vi "Generate Pattern String.vi"(10 "Options (Default)":T1, 11 "Part List":T2[](array[typedef])) -> (3 "Result":string)   [LabVIEW 2020, in "Stream.lvlib" / "URLPattern.lvclass"]
uses:
  URLPattern.lvclass
  Pattern Part.ctl
  Pattern Part Type.ctl
  Pattern Part Modifier.ctl
  Pattern String Options.ctl
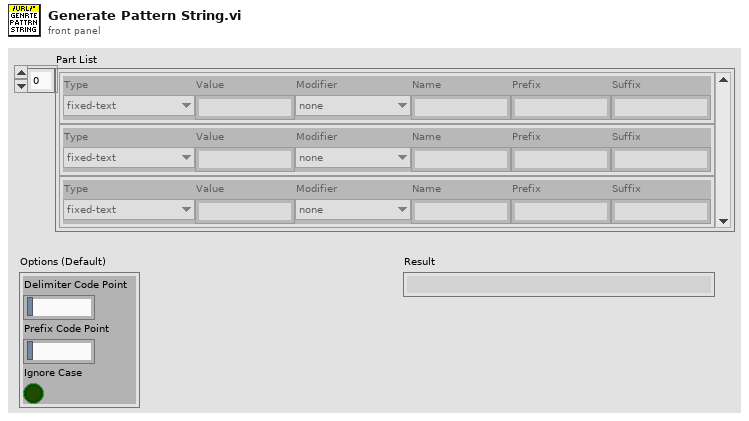
[diagram p1: front panel]
types:
  T1 = typedef "Stream.lvlib/URLPattern.lvclass/Pattern String Options.ctl" = cluster{"Delimiter Code Point":string, "Prefix Code Point":string, "Ignore Case":bool}
  T2 = typedef "Stream.lvlib/URLPattern.lvclass/Pattern Part.ctl" = cluster{"Type":T3, "Value":string, "Modifier":T4, "Name":string, "Prefix":string, "Suffix":string}
  T3 = typedef "Stream.lvlib/URLPattern.lvclass/Pattern Part Type.ctl" = enum16{"fixed-text", "regexp", "segment-wildcard", "full-wildcard"}
  T4 = typedef "Stream.lvlib/URLPattern.lvclass/Pattern Part Modifier.ctl" = enum16{"none", "optional", "zero-or-more", "one-or-more"}
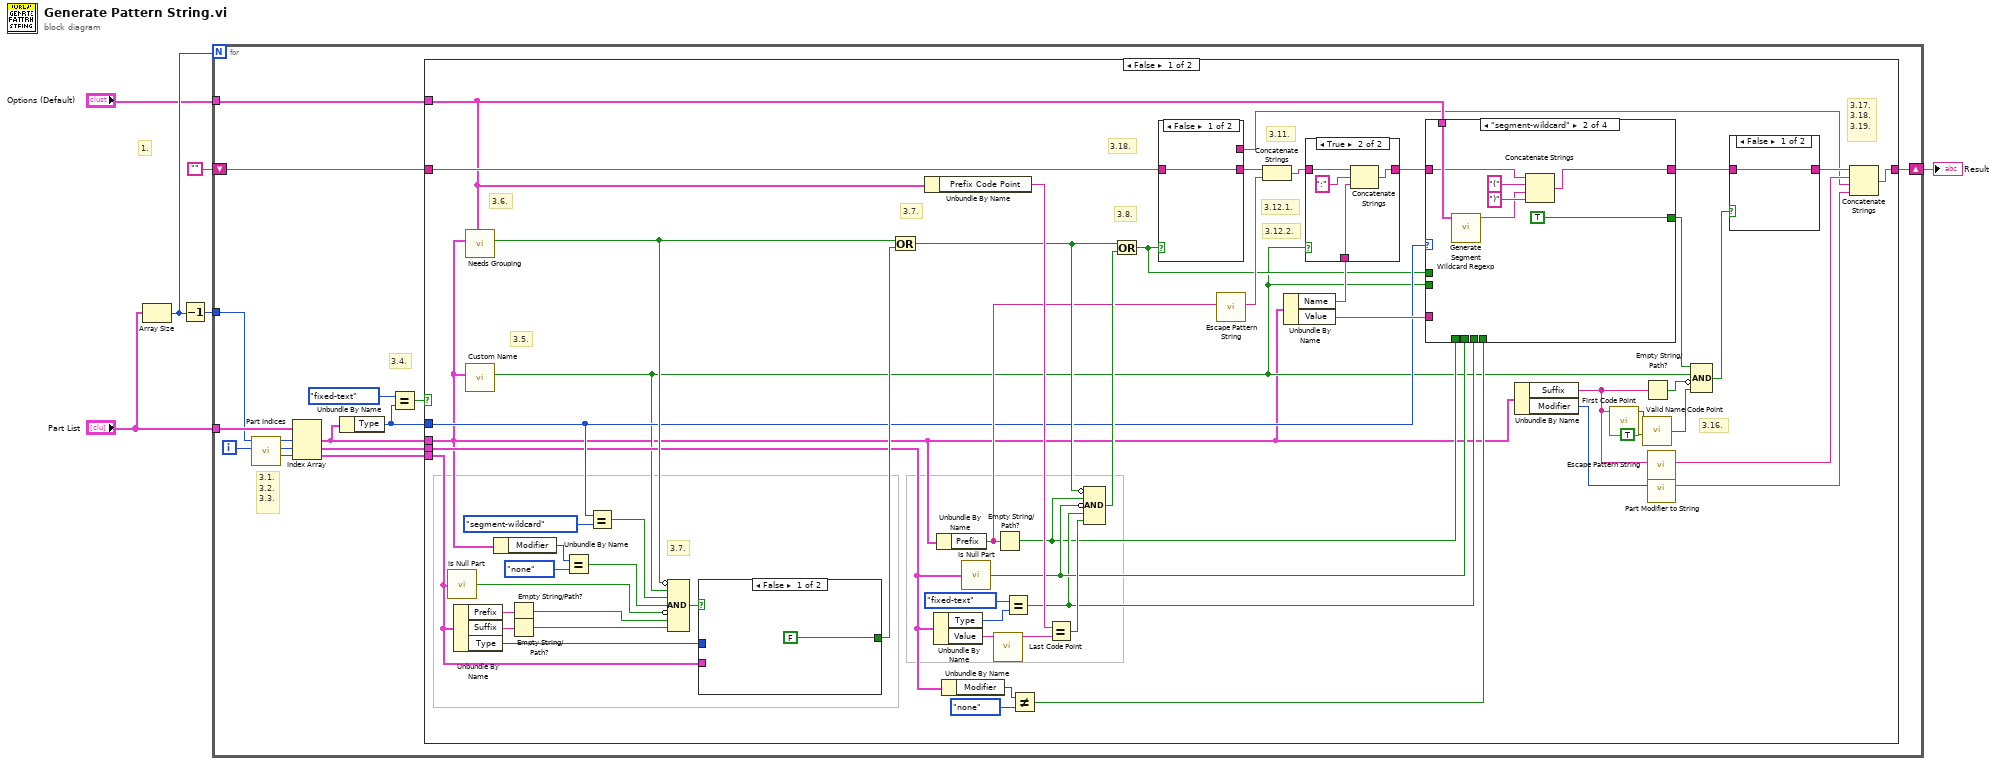
[diagram p0: block diagram]
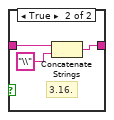
[diagram p2: hidden frame]
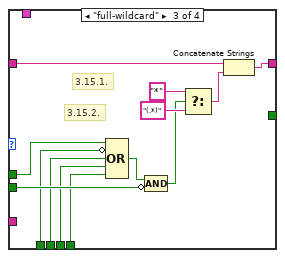
[diagram p4: hidden frame]
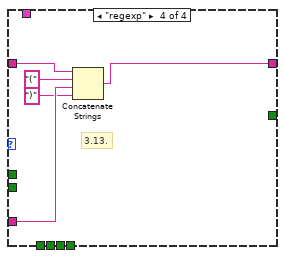
[diagram p5: hidden frame]
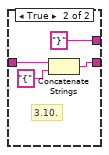
[diagram p7: hidden frame]
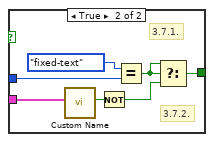
[diagram p8: hidden frame]
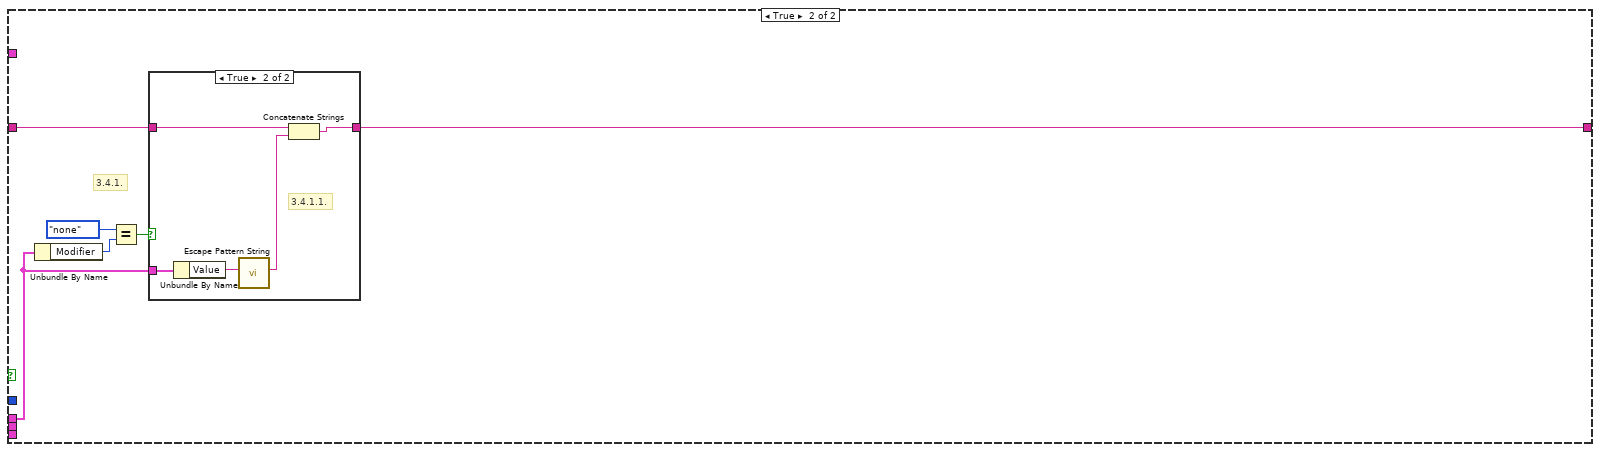
[diagram p9: hidden frame]
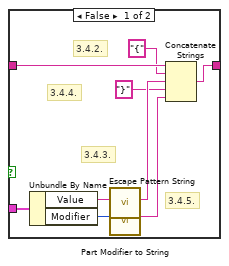
[diagram p10: hidden frame]
diagram:
  # "1."
  n1 = Array Size(array="Part List") -> (size(s)=w4:i32)
  n2 = Decrement(x=w4) -> (x-1=w3:i32)
  n3 = for {
    N: w4 -> [_]
    shift-right: [w8] -> w1
    shift-left: "" -> [w9]
    tunnel: "Part List" -> [w21]
    tunnel: w3 -> [w16]
    tunnel: "Options (Default)" -> [w10]
    i -> [w17]
    # "3.4."
    # "3.1.\n3.2.\n3.3."
    n4 = call "Part Indices.vi"("i"=w17, "Last Index"=w16) -> ("Next Index"=w18:i32, "Prev Index"=w19:i32, "Index"=w20:i32)  [unwired: 7 in]
    n5 = Index Array(array=w21, index #1=w20, index #2=w19, index #3=w18) -> (element #1=w13:T2, element #2=w12:T2, element #3=w11:T2)
    n6 = Unbundle By Name(w13) -> ("Type"=w7:T3)
    n7 = Equal?(x=Pattern_Part_Type."fixed-text", y=w7) -> (x = y?=w14:bool)
    n8 = case shown="False" w14 {
      tunnel: w13 -> [w35 w129]
      tunnel: w12 -> [w43 _]
      tunnel: w11 -> [w64 _]
      tunnel: w10 -> [w46 _]
      tunnel: w9 -> [w56 w128]
      tunnel: [w22 w127] -> w8
      tunnel: w7 -> [w47 _]
      frame False {
        # "3.18."
        # "3.17.\n3.18.\n3.19."
        # "3.16."
        # "3.12.2."
        # "3.12.1."
        # "3.11."
        # "3.8."
        # "3.7."
        # "3.7."
        # "3.6."
        # "3.5."
        n9 = call "Is Null Part.vi"("Pattern Part"=w64) -> ("Null Part"=w71:bool)
        n10 = Unbundle By Name(w64) -> ("Prefix"=w77:string, "Suffix"=w76:string, "Type"=w67:T3)
        n11 = call "Needs Grouping.vi"("Pattern String Options"=w46, "Pattern Part"=w35) -> ("Needs Grouping"=w66:bool)  [unwired: 9 in]
        n12 = call "Custom Name.vi"("Pattern Part"=w35) -> ("Custom Name?"=w36:bool)  [unwired: 10 in]
        n13 = Unbundle By Name(w35) -> ("Modifier"=w74:T4)
        n14 = Empty String/Path?(string/path=w77) -> (empty?=w70:bool)
        n15 = Empty String/Path?(string/path=w76) -> (empty?=w69:bool)
        n16 = Equal?(x=w74, y=Pattern_Part_Modifier."none") -> (x = y?=w72:bool)
        n17 = Equal?(x=w47, y=Pattern_Part_Type."segment-wildcard" ("x")) -> (x = y?=w48:bool)
        n18 = Compound Arithmetic op=AND(invert w66, w36, w48, w72, invert w71, w70, w69) -> (w68:bool)
        n19 = case shown="False" w68 {
          tunnel: w67 -> [_ w126]
          tunnel: w64 -> [_ w125]
          tunnel: [FALSE w120] -> w65
          frame False {
          }
          frame True {
            # "3.7.2."
            # "3.7.1."
            n20 = call "Custom Name.vi"("Pattern Part"=w125) -> ("Custom Name?"=w122:bool)  [unwired: 10 in]
            n21 = Not(x=w122) -> (.not. x?=w121:bool)
            n22 = Equal?(x=Pattern_Part_Type."fixed-text" ("y"), y=w126) -> (x = y?=w123:bool)
            n23 = Select(t=w123, s=w123, f=w121) -> (s? t:f=w120:bool)
          }
        }
        n24 = Or(x=w66, y=w65) -> (x .or. y?=w58:bool)
        n25 = Unbundle By Name(w46) -> ("Prefix Code Point"=w78:string)
        n26 = Unbundle By Name(w43) -> ("Type"=w63:T3, "Value"=w61:string)
        n27 = Unbundle By Name(w35) -> ("Prefix"=w55:string)
        n28 = Unbundle By Name(w43) -> ("Modifier"=w42:T4)
        n29 = call "Is Null Part.vi"("Pattern Part"=w43) -> ("Null Part"=w45:bool)
        n30 = call "Last Code Point.vi"("String"=w61) -> ("Last Code Point"=w60:string)  [unwired: 10 in]
        n31 = Empty String/Path?(string/path=w55) -> (empty?=w38:bool)
        n32 = Equal?(x=Pattern_Part_Type."fixed-text", y=w63) -> (x = y?=w44:bool)
        n33 = Not Equal?(x=w42, y=Pattern_Part_Modifier."none") -> (x != y?=w40:bool)
        n34 = Equal?(x=w78, y=w60) -> (x = y?=w59:bool)
        n35 = Compound Arithmetic op=AND(invert w58, w38, invert w45, w44, w59) -> (w57:bool)
        n36 = Or(x=w58, y=w57) -> (x .or. y?=w39:bool)
        n37 = case shown="False" w39 {
          tunnel: w56 -> [w114 w118]
          tunnel: [w114 w116] -> w54
          tunnel: [_ "}" ("string")] -> w25
          frame False {
          }
          frame True {
            # "3.10."
            n38 = Concatenate Strings(w118, "{" ("string")) -> (w116:string)
          }
        }
        n39 = call "Escape Pattern String.vi"("Input"=w55) -> ("Result"=w53:string)  [unwired: 10 in]
        n40 = Concatenate Strings(w54, w53) -> (w52:string)
        n41 = Unbundle By Name(w35) -> ("Name"=w51:string, "Value"=w49:string)
        n42 = case shown="True" w36 {
          tunnel: w52 -> [w109 w113]
          tunnel: [w109 w111] -> w50
          tunnel: w51 -> [_ w110]
          frame False {
          }
          frame True {
            n43 = Concatenate Strings(w113, ":" ("string"), w110) -> (w111:string)
          }
        }
        n44 = case shown="\"segment-wildcard\"" w47 {
          tunnel: w50 -> [w83 w87 w102 w108]
          tunnel: w49 -> [_ _ _ w106]
          tunnel: [w83 w85 w98 w104] -> w30
          tunnel: w46 -> [_ w90 _ _]
          tunnel: w36 -> [_ _ w103 _]
          tunnel: w45 -> [_ _ w96 _]
          tunnel: w44 -> [_ _ w95 _]
          tunnel: w40 -> [_ _ w94 _]
          tunnel: w39 -> [_ _ w93 _]
          tunnel: w38 -> [_ _ w92 _]
          tunnel: [_ TRUE _ _] -> w37
          frame Default {
          }
          frame "segment-wildcard" {
            n45 = call "Generate Segment Wildcard Regexp.vi"("Options"=w90) -> ("Segment Wildcard Regexp"=w86:string)  [unwired: 10 in]
            n46 = Concatenate Strings(w87, "(" ("string"), w86, ")" ("string")) -> (w85:string)
          }
          frame "full-wildcard" {
            # "3.15.2."
            # "3.15.1."
            n47 = Compound Arithmetic op=OR(w93, invert w92, w96, w95, w94) -> (w91:bool)
            n48 = Compound Arithmetic op=AND(w91, invert w103) -> (w97:bool)
            n49 = Select(t="*", s=w97, f="(.*)") -> (s? t:f=w99:string)
            n50 = Concatenate Strings(w102, w99) -> (w98:string)
          }
          frame "regexp" {
            # "3.13."
            n51 = Concatenate Strings(w108, "(" ("string"), w106, ")" ("string")) -> (w104:string)
          }
        }
        n52 = Unbundle By Name(w35) -> ("Suffix"=w28:string, "Modifier"=w24:T4)
        n53 = call "First Code Point.vi"("String"=w28) -> ("First Code Point"=w33:u32)  [unwired: 10 in]
        n54 = call "Valid Name Code Point.vi"("First"=TRUE, "Code Point"=w33) -> ("Valid?"=w29:bool)  [unwired: 2 in]
        n55 = Empty String/Path?(string/path=w28) -> (empty?=w34:bool)
        n56 = call "Escape Pattern String.vi"("Input"=w28) -> ("Result"=w26:string)  [unwired: 10 in]
        n57 = call "Part Modifier to String.vi"("Pattern Part Modifier"=w24) -> ("String"=w23:string)  [unwired: 10 in]
        n58 = Compound Arithmetic op=AND(w37, w36, invert w34, w29) -> (w31:bool)
        n59 = case shown="False" w31 {
          tunnel: w30 -> [w79 w82]
          tunnel: [w79 w80] -> w27
          frame False {
          }
          frame True {
            # "3.16."
            n60 = Concatenate Strings(w82, "\\" ("string")) -> (w80:string)
          }
        }
        n61 = Concatenate Strings(w27, w26, w25, w23) -> (w22:string)
      }
      frame True {
        # "3.4.1."
        n62 = Unbundle By Name(w129) -> ("Modifier"=w132:T4)
        n63 = Equal?(x=Pattern_Part_Modifier."none", y=w132) -> (x = y?=w130:bool)
        n64 = case shown="True" w130 {
          tunnel: w129 -> [w139 w146]
          tunnel: w128 -> [w141 w144]
          tunnel: [w133 w142] -> w127
          frame False {
            # "3.4.5."
            # "3.4.4."
            # "3.4.3."
            # "3.4.2."
            n65 = Unbundle By Name(w139) -> ("Value"=w138:string, "Modifier"=w135:T4)
            n66 = call "Escape Pattern String.vi"("Input"=w138) -> ("Result"=w137:string)  [unwired: 10 in]
            n67 = call "Part Modifier to String.vi"("Pattern Part Modifier"=w135) -> ("String"=w134:string)  [unwired: 10 in]
            n68 = Concatenate Strings(w141, "{" ("string"), w137, "}" ("string"), w134) -> (w133:string)
          }
          frame True {
            # "3.4.1.1."
            n69 = Unbundle By Name(w146) -> ("Value"=w145:string)
            n70 = call "Escape Pattern String.vi"("Input"=w145) -> ("Result"=w143:string)  [unwired: 10 in]
            n71 = Concatenate Strings(w144, w143) -> (w142:string)
          }
        }
      }
    }
  }
  "Result" <- w1
